vi "Address2Coordinate.vi"(1 "Address":string) -> (0 "Coordinate":i32[](array[numeric]))   [LabVIEW 2013, in "XCel Report Engine.lvlib"]
doc: "Converts an Excel A1 cell address to zero-based row and column coordinates.\n\nFor example, A1 returns row 0 and column 0, while O13 returns row 12 and column 14.\n\nCell addresses are case-insensitive and may use absolute notation, such as $O$13.\n\nAn error is returned if the address is empty, malformed, represents a range, or exceeds the Excel worksheet limits.\n\nThis conversion does not require an open report session."
uses:
  XCel Report Engine.lvlib
  C:/Users/m.santucci/Documents/ChatGPT/LV_REPORT_ENGINE/LV/DotNet/XCelReportEngine.dll
  LV/DotNet/XCelReportEngine.dll
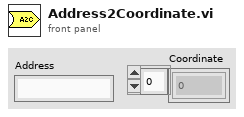
[diagram p1: front panel]
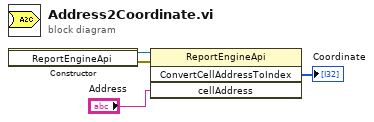
[diagram p0: block diagram]
diagram:
  n1 = constructor class="ReportEngineApi"() -> (reference out=w4:refnum<k24>, error out=w3:errorcluster)  [unwired: 3 in, 1 out]
  n2 = invoke class="ReportEngineApi" method="ConvertCellAddressToIndex"(reference=w4, error in=w3, "cellAddress"="Address") -> ("ConvertCellAddressToIndex"=→"Coordinate":i32[])  [unwired: 1 in, 3 out]
